vi "DAQ.vi"() -> (0 "Error Out":errorcluster)   [LabVIEW 2017]
uses:
  <vilib>/dex/Flush And Wait Empty Condition.ctl
  <vilib>/Platform/TimedLoop/XDataNode/timing_clust.ctl
  <vilib>/Platform/TimedLoop/XDataNode/nitl_modes.ctl
  <vilib>/Platform/TimedLoop/XDataNode/wakeup.ctl
  <vilib>/DAQmx/read.llb/DAQmx Read (Analog 1D DBL NChan 1Samp).vi
  <vilib>/DAQmx/miscellaneous.llb/DAQmx Fill In Error Info.vi
  <vilib>/Platform/TimedLoop/XDataNode/XDataNode.xnode
  <vilib>/Platform/TimedLoop/XDataNode/XDNodeRunTimeDep.lvlib
  <resource>/objmgr/ni.dex.rc
panel:
  out "Producer Loop Time":i64
  out "Consumer Loop Time":u32
  in  "Error In":errorcluster
  out "Time":dbl
  out "Available Elements for Writing":i32
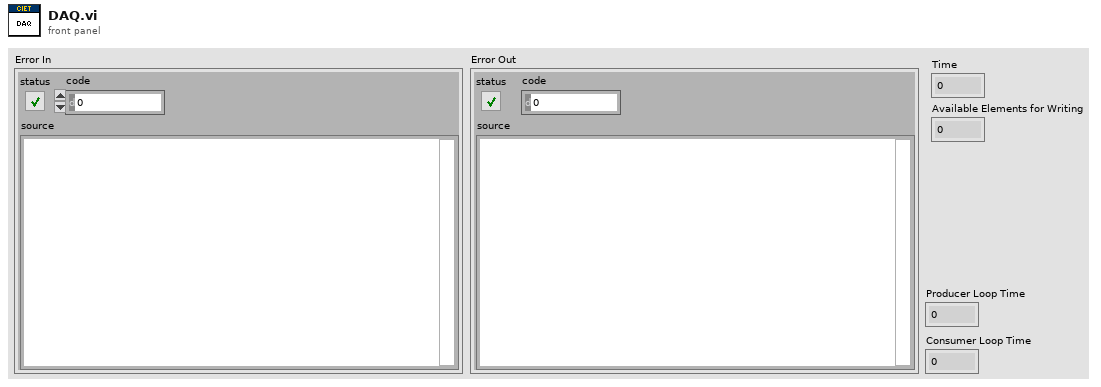
[diagram p1: front panel]
types:
  T1 = typedef "Flush And Wait Empty Condition.ctl" = u8
  T2 = typedef "XDNodeRunTimeDep.lvlib/timing_clust.ctl" = cluster{"Expected End [f-1]":u64, "Actual End [f-1]":u64, "Finished Late? [f-1]":bool, "Expected End [i-1]":u64, "Actual End [i-1]":u64, "Finished Late? [i-1]":bool, "Expected Start [i]":u64, "Actual Start [i]":u64, "Expected Start [f]":u64, "Actual Start [f]":u64, "Source Name":string, "Structure Name":string, "Period":i64, "Deadline":i64, "Offset":i64, "Start":i64, "Priority":i32, "Timeout":i32, "Mode":T3, "Wakeup Reason":T4, "Error":errorcluster, "Source Type":string, "Secondary Source Type":string, "Global End Time":u64, "Global Start Time":u64, "Frame Duration":u64, "Iteration Duration":u64, "Assigned CPU":i32, "I/O Scan Engine Mode":u32}
  T3 = typedef "XDNodeRunTimeDep.lvlib/nitl_modes.ctl" = enum32{"No Change", "Process missed periods, maintain original phase", "Discard missed periods, maintain original phase", "Process missed periods, ignore original phase", "Discard missed periods, ignore original phase"}
  T4 = typedef "XDNodeRunTimeDep.lvlib/wakeup.ctl" = enum32{"Normal", "Aborted", "Asynchronous wakeup", "Timing source error", "Timed loop error", "Timeout"}
  T5 = cluster{"[0]":sgl, "[1]":sgl, "[2]":sgl, "[3]":sgl, "[4]":sgl, "[5]":sgl, "[6]":sgl, "[7]":sgl, "[8]":sgl, "[9]":sgl, "[10]":sgl, "[11]":sgl, "[12]":sgl, "[13]":sgl, "[14]":sgl, "[15]":sgl, "[16]":sgl, "[17]":sgl, "[18]":sgl, "[19]":sgl, "[20]":sgl, "[21]":sgl, "[22]":sgl, "[23]":sgl, "[24]":sgl, "[25]":sgl, "[26]":sgl, "[27]":sgl, "[28]":sgl, "[29]":sgl, "[30]":sgl, "[31]":sgl, "[32]":sgl, "[33]":sgl, "[34]":sgl, "[35]":sgl, "[36]":sgl, "[37]":sgl, "[38]":sgl, "[39]":sgl, "[40]":sgl, "[41]":sgl, "[42]":sgl, "[43]":sgl, "[44]":sgl, "[45]":sgl, "[46]":sgl, "[47]":sgl, "[48]":sgl, "[49]":sgl, "[50]":sgl, "[51]":sgl, "[52]":sgl, "[53]":sgl, "[54]":sgl, "[55]":sgl, "[56]":sgl}
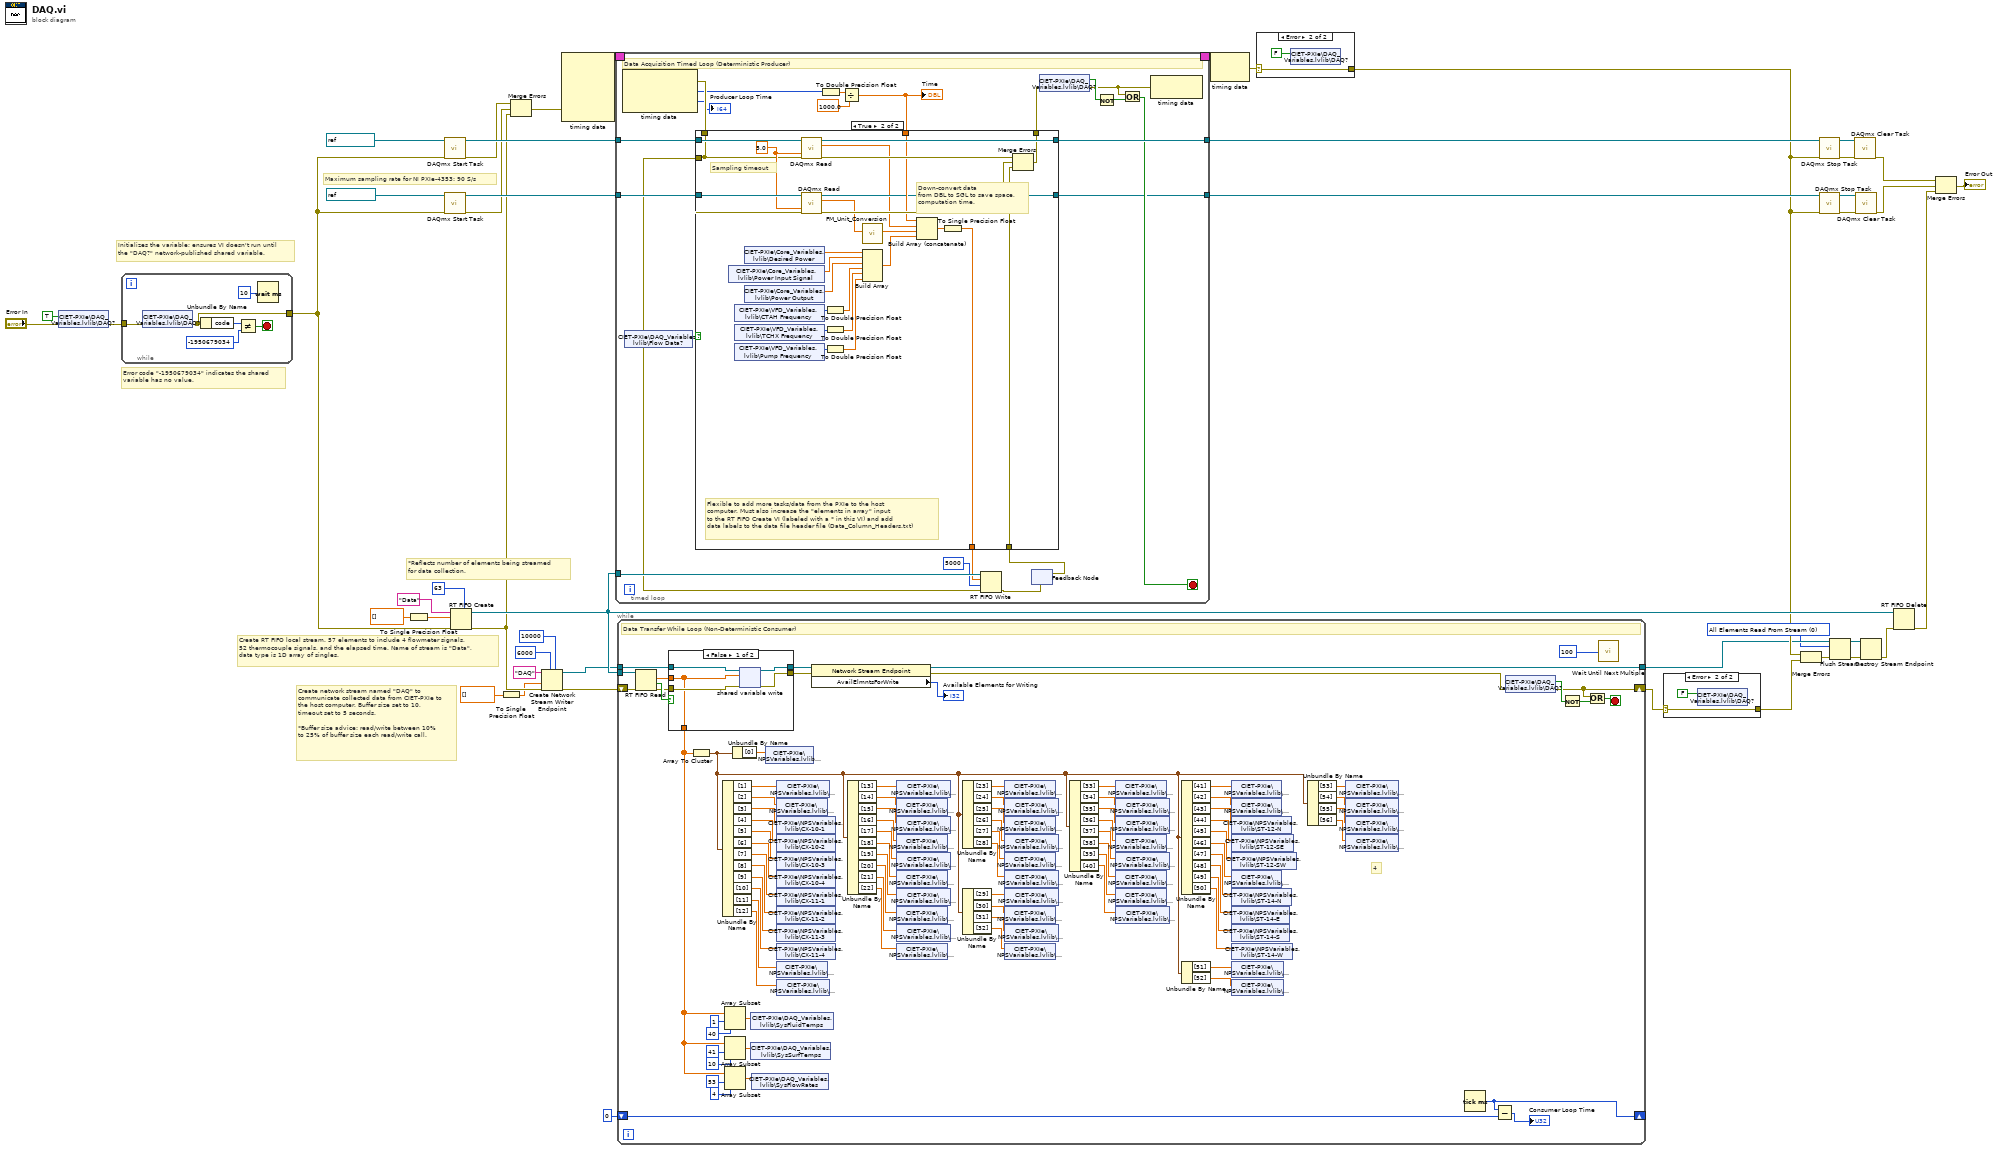
[diagram p0: block diagram]
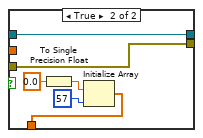
[diagram p4: hidden frame]
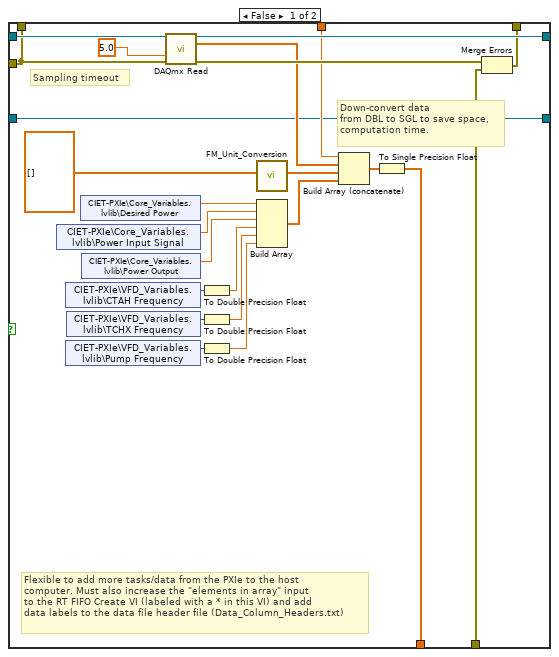
[diagram p5: hidden frame]
diagram:
  w3 = T1 0 items=["All Elements Read From Stream", "All Elements Available for Reading"] ("wait condition")
  # "*Reflects number of elements being streamed\nfor data collection."
  # "Create RT FIFO local stream. 57 elements to include 4 flowmeter signals,\n52 thermocouple signals, and the elapsed time. Name of stream is \"Data\",\ndata type is 1D array of singles."
  # "Create network stream named \"DAQ\" to communicate collected data from CIET-PXIe to the host computer. Buffer size set to 10, timeout set to 5 seconds. \n\n*Buffer size advice: read/write between 10%\nto 25% of buffer size each read/write call."
  # "Maximum sampling rate for NI PXIe-4353: 90 S/s"
  # "Initializes the variable; ensures VI doesn't run until\nthe \"DAQ?\" network-published shared variable."
  # "Error code \"-1950679034\" indicates the shared\nvariable has no value."
  n1 = shared-variable "CIET-PXIe\\DAQ_Variables.lvlib\\DAQ?"(TRUE ("Active?"), error in="Error In") -> (error out=w23:errorcluster)
  n2 = while {
    tunnel: w23 -> [w52]
    tunnel: [w51] -> w22
    stop <- w48 stop-if-true
    n3 = shared-variable "CIET-PXIe\\DAQ_Variables.lvlib\\DAQ?"(error in=w52) -> (error out=w51:errorcluster)  [unwired: 1 out]
    n4 = Unbundle By Name(w51) -> ("code"=w50:i32)
    n5 = Not Equal?(x=w50, y=-1950679034) -> (x != y?=w48:bool)
    n6 = Wait (ms)(milliseconds to wait=u32 10) -> ()  [unwired: 1 out]
  }
  n7 = To Single Precision Float(number=dbl[] []) -> (single precision float=w33:sgl[])
  n8 = call <vilib>:"DAQmx Start Task.vi"("task/channels in"=refnum<k21> "CIET-TC", "error in"=w22) -> ("task out"=w43:refnum<k21>, "error out"=w27:errorcluster)  [unwired: 12 in]
  n9 = call <vilib>:"DAQmx Start Task.vi"("task/channels in"=refnum<k21> "CIET-FM", "error in"=w22) -> ("task out"=w42:refnum<k21>, "error out"=w28:errorcluster)  [unwired: 12 in]
  n10 = RT FIFO Create(0:"Data" ("name (unnamed)"), 1:w33, 3:w22, 6:u32 63 ("elements in array (1)")) -> (8:w26:refnum<k33>, 11:w18:errorcluster)  [unwired: 4 in, 1 out]
  n11 = To Single Precision Float(number=dbl[] []) -> (single precision float=w8:sgl[])
  n12 = Merge Errors(w27, w28, w18) -> (w29:errorcluster)
  n13 = Create Network Stream Writer Endpoint(5:10000 ("timeout in ms (-1)"), 7:6000 ("writer buffer size"), 8:w18, 9:w8, 11:"DAQ" ("writer name")) -> (0:w19:errorcluster, 3:w17:refnum<k21>)  [unwired: 2 in]
  n14 = node-c288(w29) -> (w47:T2)  [unwired: 4 in]
  n15 = timed-loop {
    timing: w47 -> [_]
    timing-out: [_] -> w46
    tunnel: w26 -> [w72]
    tunnel: w43 -> [w75]
    tunnel: [w73] -> w37
    tunnel: w42 -> [w74]
    tunnel: [w60] -> w36
    stop <- w67 stop-if-true
    # "Data Acquisition Timed Loop (Deterministic Producer)"
    n16 = node-c288() -> (w70:errorcluster, w61:i64, →"Producer Loop Time":i64)  [unwired: 1 in]
    n17 = shared-variable "CIET-PXIe\\DAQ_Variables.lvlib\\Flow Data?"() -> (w55:bool)  [unwired: 1 in, 1 out]
    n18 = To Double Precision Float(number=w61) -> (double precision float=w64:dbl)
    n19 = Divide(x=w64, y=1000.0) -> (x/y=w63:dbl)
    "Time" <- w63
    n20 = feedback #1() -> (w56:errorcluster)  [unwired: 1 in]
    n21 = case shown="True" w55 {
      tunnel: w75 -> [w99 w125]
      tunnel: w74 -> [w79 w124]
      tunnel: [w97 w122] -> w73
      tunnel: [w95 w120] -> w58
      tunnel: w70 -> [w76 w100]
      tunnel: w56 -> [w77 w117]
      tunnel: [w93 w116] -> w66
      tunnel: w63 -> [w92 w115]
      tunnel: [w79 w114] -> w60
      tunnel: [w76 w100] -> w54
      frame False {
        # "Flexible to add more tasks/data from the PXIe to the host \ncomputer. Must also increase the \"elements in array\" input \nto the RT FIFO Create VI (labeled with a * in this VI) and add\ndata labels to the data file header file (Data_Column_Headers.txt)"
        # "Down-convert data\nfrom DBL to SGL to save space,\ncomputation time."
        # "Sampling timeout"
        n22 = shared-variable "CIET-PXIe\\Core_Variables.lvlib\\Power Input Signal"() -> (w82:dbl)  [unwired: 1 in, 1 out]
        n23 = shared-variable "CIET-PXIe\\VFD_Variables.lvlib\\CTAH Frequency"() -> (w84:u16)  [unwired: 1 in, 1 out]
        n24 = shared-variable "CIET-PXIe\\VFD_Variables.lvlib\\Pump Frequency"() -> (w86:u16)  [unwired: 1 in, 1 out]
        n25 = shared-variable "CIET-PXIe\\VFD_Variables.lvlib\\TCHX Frequency"() -> (w85:u16)  [unwired: 1 in, 1 out]
        n26 = shared-variable "CIET-PXIe\\Core_Variables.lvlib\\Desired Power"() -> (w81:dbl)  [unwired: 1 in, 1 out]
        n27 = shared-variable "CIET-PXIe\\Core_Variables.lvlib\\Power Output"() -> (w83:dbl)  [unwired: 1 in, 1 out]
        n28 = call-poly <vilib>:"DAQmx Read.vi"("task/channels in"=w99, "timeout"=5.0, "error in"=w76) -> ("task out"=w97:refnum<k21>, "data"=w91:dbl[], "error out"=w94:errorcluster)  [unwired: 10 in]
        n29 = To Double Precision Float(number=w84) -> (double precision float=w87:dbl)
        n30 = To Double Precision Float(number=w85) -> (double precision float=w88:dbl)
        n31 = To Double Precision Float(number=w86) -> (double precision float=w89:dbl)
        n32 = call "FM_Unit_Conversion.vi"("Input Array [A]"=dbl[] []) -> ("Output Array [kg/h]"=w90:dbl[])  [unwired: 10 in]
        n33 = Build Array(w81, w82, w83, w87, w88, w89) -> (w80:dbl[])
        n34 = Build Array (concatenate)(w92, w91, w90, w80) -> (w96:dbl[])
        n35 = To Single Precision Float(number=w96) -> (single precision float=w95:sgl[])
        n36 = Merge Errors(w94, w77) -> (w93:errorcluster)
      }
      frame True {
        w123 = 5.0 ("timeout")
        # "Flexible to add more tasks/data from the PXIe to the host \ncomputer. Must also increase the \"elements in array\" input \nto the RT FIFO Create VI (labeled with a * in this VI) and add\ndata labels to the data file header file (Data_Column_Headers.txt)"
        # "Down-convert data\nfrom DBL to SGL to save space,\ncomputation time."
        # "Sampling timeout"
        n37 = shared-variable "CIET-PXIe\\Core_Variables.lvlib\\Power Input Signal"() -> (w103:dbl)  [unwired: 1 in, 1 out]
        n38 = shared-variable "CIET-PXIe\\VFD_Variables.lvlib\\CTAH Frequency"() -> (w105:u16)  [unwired: 1 in, 1 out]
        n39 = shared-variable "CIET-PXIe\\VFD_Variables.lvlib\\Pump Frequency"() -> (w107:u16)  [unwired: 1 in, 1 out]
        n40 = shared-variable "CIET-PXIe\\VFD_Variables.lvlib\\TCHX Frequency"() -> (w106:u16)  [unwired: 1 in, 1 out]
        n41 = shared-variable "CIET-PXIe\\Core_Variables.lvlib\\Desired Power"() -> (w102:dbl)  [unwired: 1 in, 1 out]
        n42 = shared-variable "CIET-PXIe\\Core_Variables.lvlib\\Power Output"() -> (w104:dbl)  [unwired: 1 in, 1 out]
        n43 = call-poly <vilib>:"DAQmx Read.vi"("task/channels in"=w125, "timeout"=w123, "error in"=w100) -> ("task out"=w122:refnum<k21>, "data"=w113:dbl[], "error out"=w118:errorcluster)  [unwired: 10 in]
        n44 = call-poly <vilib>:"DAQmx Read.vi"("task/channels in"=w124, "timeout"=w123, "error in"=w100) -> ("task out"=w114:refnum<k21>, "data"=w111:dbl[], "error out"=w119:errorcluster)  [unwired: 10 in]
        n45 = To Double Precision Float(number=w105) -> (double precision float=w108:dbl)
        n46 = To Double Precision Float(number=w106) -> (double precision float=w109:dbl)
        n47 = To Double Precision Float(number=w107) -> (double precision float=w110:dbl)
        n48 = call "FM_Unit_Conversion.vi"("Input Array [A]"=w111) -> ("Output Array [kg/h]"=w112:dbl[])  [unwired: 10 in]
        n49 = Build Array(w102, w103, w104, w108, w109, w110) -> (w101:dbl[])
        n50 = Build Array (concatenate)(w115, w113, w112, w101) -> (w121:dbl[])
        n51 = To Single Precision Float(number=w121) -> (single precision float=w120:sgl[])
        n52 = Merge Errors(w118, w119, w117) -> (w116:errorcluster)
      }
    }
    n53 = RT FIFO Write(0:w72, 1:w58, 2:5000 ("timeout in ms (0)"), 3:w54) -> (11:w57:errorcluster)  [unwired: 1 in, 3 out]
    n54 = feedback-in #1(w57) -> ()
    n55 = shared-variable "CIET-PXIe\\DAQ_Variables.lvlib\\DAQ?"(error in=w66) -> (w69:bool, error out=w65:errorcluster)
    n56 = Not(x=w69) -> (.not. x?=w68:bool)
    n57 = Or(x=w65, y=w68) -> (x .or. y?=w67:bool)
    n58 = node-c288(w65) -> ()  [unwired: 1 out]
  }
  n59 = while {
    tunnel: w26 -> [w219]
    shift-right: [w208] -> w20
    shift-left: w19 -> [w218]
    tunnel: w17 -> [w210]
    tunnel: [w205] -> w10
    shift-right: [w145] -> _
    shift-left: u32 0 ("millisecond timer value") -> [w144]
    stop <- w211 stop-if-true
    # "4"
    # "Data Transfer While Loop (Non-Deterministic Consumer)"
    n60 = RT FIFO Read(0:w219, 3:w218) -> (9:w215:sgl[], 10:w216:bool, 11:w214:errorcluster)  [unwired: 2 in, 2 out]
    n61 = case shown="False" w216 {
      tunnel: w215 -> [w220 _]
      tunnel: w214 -> [w224 w230]
      tunnel: [w223 w230] -> w207
      tunnel: w210 -> [w222 w229]
      tunnel: [w221 w229] -> w206
      tunnel: [w220 w225] -> w136
      frame False {
        n62 = shared-variable-write(w222, w224, w220) -> (w221:refnum<k21>, w223:errorcluster)  [unwired: 1 in, 1 out]
      }
      frame True {
        n63 = To Single Precision Float(number=sgl 0.0) -> (single precision float=w228:sgl)
        n64 = Initialize Array(w228, 57 ("dimension size")) -> (w225:sgl[])
      }
    }
    n65 = Array To Cluster(array=w136) -> (cluster=w146:T5)
    n66 = Unbundle By Name(w146) -> ("[1]"=w202:sgl, "[2]"=w201:sgl, "[3]"=w200:sgl, "[4]"=w199:sgl, "[5]"=w198:sgl, "[6]"=w197:sgl, "[7]"=w196:sgl, "[8]"=w195:sgl, "[9]"=w194:sgl, "[10]"=w193:sgl, "[11]"=w192:sgl, "[12]"=w191:sgl)
    n67 = Array Subset(array=w136, index=1, length=40) -> (w140:sgl[])
    n68 = Array Subset(array=w136, index=41, length=10) -> (w138:sgl[])
    n69 = Array Subset(array=w136, index=53, length=4) -> (w133:sgl[])
    n70 = Unbundle By Name(w146) -> ("[0]"=w203:sgl)
    n71 = shared-variable "CIET-PXIe\\DAQ_Variables.lvlib\\SysFluidTemps"(w140) -> ()  [unwired: 1 in, 1 out]
    n72 = shared-variable "CIET-PXIe\\DAQ_Variables.lvlib\\SysSurfTemps"(w138) -> ()  [unwired: 1 in, 1 out]
    n73 = shared-variable "CIET-PXIe\\DAQ_Variables.lvlib\\SysFlowRates"(w133) -> ()  [unwired: 1 in, 1 out]
    n74 = shared-variable "CIET-PXIe\\NPSVariables.lvlib\\Time"(w203) -> ()  [unwired: 1 in, 1 out]
    n75 = shared-variable "CIET-PXIe\\NPSVariables.lvlib\\WT-10"(w202) -> ()  [unwired: 1 in, 1 out]
    n76 = shared-variable "CIET-PXIe\\NPSVariables.lvlib\\BT-11"(w201) -> ()  [unwired: 1 in, 1 out]
    n77 = shared-variable "CIET-PXIe\\NPSVariables.lvlib\\CX-10-1"(w200) -> ()  [unwired: 1 in, 1 out]
    n78 = shared-variable "CIET-PXIe\\NPSVariables.lvlib\\CX-10-2"(w199) -> ()  [unwired: 1 in, 1 out]
    n79 = shared-variable "CIET-PXIe\\NPSVariables.lvlib\\CX-10-3"(w198) -> ()  [unwired: 1 in, 1 out]
    n80 = shared-variable "CIET-PXIe\\NPSVariables.lvlib\\CX-10-4"(w197) -> ()  [unwired: 1 in, 1 out]
    n81 = shared-variable "CIET-PXIe\\NPSVariables.lvlib\\CX-11-1"(w196) -> ()  [unwired: 1 in, 1 out]
    n82 = shared-variable "CIET-PXIe\\NPSVariables.lvlib\\CX-11-2"(w195) -> ()  [unwired: 1 in, 1 out]
    n83 = shared-variable "CIET-PXIe\\NPSVariables.lvlib\\CX-11-3"(w194) -> ()  [unwired: 1 in, 1 out]
    n84 = shared-variable "CIET-PXIe\\NPSVariables.lvlib\\CX-11-4"(w193) -> ()  [unwired: 1 in, 1 out]
    n85 = shared-variable "CIET-PXIe\\NPSVariables.lvlib\\BT-12"(w192) -> ()  [unwired: 1 in, 1 out]
    n86 = shared-variable "CIET-PXIe\\NPSVariables.lvlib\\WT-13"(w191) -> ()  [unwired: 1 in, 1 out]
    n87 = property class="Network Stream Endpoint"(reference=w206, error in=w207) -> (reference out=w205:refnum<k21>, error out=w204:errorcluster, "AvailElmntsForWrite"=→"Available Elements for Writing":i32)
    n88 = Unbundle By Name(w146) -> ("[13]"=w190:sgl, "[14]"=w189:sgl, "[15]"=w188:sgl, "[16]"=w187:sgl, "[17]"=w186:sgl, "[18]"=w185:sgl, "[19]"=w184:sgl, "[20]"=w183:sgl, "[21]"=w182:sgl, "[22]"=w181:sgl)
    n89 = shared-variable "CIET-PXIe\\NPSVariables.lvlib\\WT-20"(w190) -> ()  [unwired: 1 in, 1 out]
    n90 = shared-variable "CIET-PXIe\\NPSVariables.lvlib\\BT-21"(w189) -> ()  [unwired: 1 in, 1 out]
    n91 = shared-variable "CIET-PXIe\\NPSVariables.lvlib\\WT-22"(w188) -> ()  [unwired: 1 in, 1 out]
    n92 = shared-variable "CIET-PXIe\\NPSVariables.lvlib\\BT-23"(w187) -> ()  [unwired: 1 in, 1 out]
    n93 = shared-variable "CIET-PXIe\\NPSVariables.lvlib\\WT-24"(w186) -> ()  [unwired: 1 in, 1 out]
    n94 = shared-variable "CIET-PXIe\\NPSVariables.lvlib\\BT-25"(w185) -> ()  [unwired: 1 in, 1 out]
    n95 = shared-variable "CIET-PXIe\\NPSVariables.lvlib\\WT-26"(w184) -> ()  [unwired: 1 in, 1 out]
    n96 = shared-variable "CIET-PXIe\\NPSVariables.lvlib\\BT-27"(w183) -> ()  [unwired: 1 in, 1 out]
    n97 = shared-variable "CIET-PXIe\\NPSVariables.lvlib\\WT-28"(w182) -> ()  [unwired: 1 in, 1 out]
    n98 = shared-variable "CIET-PXIe\\NPSVariables.lvlib\\BT-29"(w181) -> ()  [unwired: 1 in, 1 out]
    n99 = Unbundle By Name(w146) -> ("[23]"=w180:sgl, "[24]"=w179:sgl, "[25]"=w178:sgl, "[26]"=w177:sgl, "[27]"=w176:sgl, "[28]"=w175:sgl)
    n100 = Unbundle By Name(w146) -> ("[29]"=w174:sgl, "[30]"=w173:sgl, "[31]"=w172:sgl, "[32]"=w171:sgl)
    n101 = shared-variable "CIET-PXIe\\NPSVariables.lvlib\\BT-30"(w180) -> ()  [unwired: 1 in, 1 out]
    n102 = shared-variable "CIET-PXIe\\NPSVariables.lvlib\\WT-31"(w179) -> ()  [unwired: 1 in, 1 out]
    n103 = shared-variable "CIET-PXIe\\NPSVariables.lvlib\\BT-32"(w178) -> ()  [unwired: 1 in, 1 out]
    n104 = shared-variable "CIET-PXIe\\NPSVariables.lvlib\\WT-33"(w177) -> ()  [unwired: 1 in, 1 out]
    n105 = shared-variable "CIET-PXIe\\NPSVariables.lvlib\\BT-34"(w176) -> ()  [unwired: 1 in, 1 out]
    n106 = shared-variable "CIET-PXIe\\NPSVariables.lvlib\\WT-35"(w175) -> ()  [unwired: 1 in, 1 out]
    n107 = shared-variable "CIET-PXIe\\NPSVariables.lvlib\\WT-40"(w174) -> ()  [unwired: 1 in, 1 out]
    n108 = shared-variable "CIET-PXIe\\NPSVariables.lvlib\\BT-41"(w173) -> ()  [unwired: 1 in, 1 out]
    n109 = shared-variable "CIET-PXIe\\NPSVariables.lvlib\\WT-42"(w172) -> ()  [unwired: 1 in, 1 out]
    n110 = shared-variable "CIET-PXIe\\NPSVariables.lvlib\\BT-43"(w171) -> ()  [unwired: 1 in, 1 out]
    n111 = Unbundle By Name(w146) -> ("[33]"=w170:sgl, "[34]"=w169:sgl, "[35]"=w168:sgl, "[36]"=w167:sgl, "[37]"=w166:sgl, "[38]"=w165:sgl, "[39]"=w164:sgl, "[40]"=w163:sgl)
    n112 = shared-variable "CIET-PXIe\\NPSVariables.lvlib\\BT-60"(w170) -> ()  [unwired: 1 in, 1 out]
    n113 = shared-variable "CIET-PXIe\\NPSVariables.lvlib\\WT-61"(w169) -> ()  [unwired: 1 in, 1 out]
    n114 = shared-variable "CIET-PXIe\\NPSVariables.lvlib\\WT-62"(w168) -> ()  [unwired: 1 in, 1 out]
    n115 = shared-variable "CIET-PXIe\\NPSVariables.lvlib\\BT-63"(w167) -> ()  [unwired: 1 in, 1 out]
    n116 = shared-variable "CIET-PXIe\\NPSVariables.lvlib\\WT-64"(w166) -> ()  [unwired: 1 in, 1 out]
    n117 = shared-variable "CIET-PXIe\\NPSVariables.lvlib\\BT-65"(w165) -> ()  [unwired: 1 in, 1 out]
    n118 = shared-variable "CIET-PXIe\\NPSVariables.lvlib\\BT-66"(w164) -> ()  [unwired: 1 in, 1 out]
    n119 = shared-variable "CIET-PXIe\\NPSVariables.lvlib\\WT-67"(w163) -> ()  [unwired: 1 in, 1 out]
    n120 = Unbundle By Name(w146) -> ("[41]"=w162:sgl, "[42]"=w161:sgl, "[43]"=w160:sgl, "[44]"=w159:sgl, "[45]"=w158:sgl, "[46]"=w157:sgl, "[47]"=w156:sgl, "[48]"=w155:sgl, "[49]"=w154:sgl, "[50]"=w153:sgl)
    n121 = Unbundle By Name(w146) -> ("[51]"=w152:sgl, "[52]"=w151:sgl)
    n122 = shared-variable "CIET-PXIe\\NPSVariables.lvlib\\ST-10"(w162) -> ()  [unwired: 1 in, 1 out]
    n123 = shared-variable "CIET-PXIe\\NPSVariables.lvlib\\ST-11"(w161) -> ()  [unwired: 1 in, 1 out]
    n124 = shared-variable "CIET-PXIe\\NPSVariables.lvlib\\ST-12-N"(w160) -> ()  [unwired: 1 in, 1 out]
    n125 = shared-variable "CIET-PXIe\\NPSVariables.lvlib\\ST-12-SE"(w159) -> ()  [unwired: 1 in, 1 out]
    n126 = shared-variable "CIET-PXIe\\NPSVariables.lvlib\\ST-12-SW"(w158) -> ()  [unwired: 1 in, 1 out]
    n127 = shared-variable "CIET-PXIe\\NPSVariables.lvlib\\ST-13"(w157) -> ()  [unwired: 1 in, 1 out]
    n128 = shared-variable "CIET-PXIe\\NPSVariables.lvlib\\ST-14-N"(w156) -> ()  [unwired: 1 in, 1 out]
    n129 = shared-variable "CIET-PXIe\\NPSVariables.lvlib\\ST-14-E"(w155) -> ()  [unwired: 1 in, 1 out]
    n130 = shared-variable "CIET-PXIe\\NPSVariables.lvlib\\ST-14-S"(w154) -> ()  [unwired: 1 in, 1 out]
    n131 = shared-variable "CIET-PXIe\\NPSVariables.lvlib\\ST-14-W"(w153) -> ()  [unwired: 1 in, 1 out]
    n132 = shared-variable "CIET-PXIe\\NPSVariables.lvlib\\AT-01"(w152) -> ()  [unwired: 1 in, 1 out]
    n133 = shared-variable "CIET-PXIe\\NPSVariables.lvlib\\AT-02"(w151) -> ()  [unwired: 1 in, 1 out]
    n134 = Unbundle By Name(w146) -> ("[53]"=w150:sgl, "[54]"=w149:sgl, "[55]"=w148:sgl, "[56]"=w147:sgl)
    n135 = shared-variable "CIET-PXIe\\NPSVariables.lvlib\\FM-20"(w150) -> ()  [unwired: 1 in, 1 out]
    n136 = shared-variable "CIET-PXIe\\NPSVariables.lvlib\\FM-30"(w149) -> ()  [unwired: 1 in, 1 out]
    n137 = shared-variable "CIET-PXIe\\NPSVariables.lvlib\\FM-40"(w148) -> ()  [unwired: 1 in, 1 out]
    n138 = shared-variable "CIET-PXIe\\NPSVariables.lvlib\\FM-60"(w147) -> ()  [unwired: 1 in, 1 out]
    n139 = Tick Count (ms)() -> (millisecond timer value=w145:u32)
    n140 = Subtract(x=w145, y=w144) -> (x-y=→"Consumer Loop Time":u32)
    n141 = shared-variable "CIET-PXIe\\DAQ_Variables.lvlib\\DAQ?"(error in=w204) -> (w213:bool, error out=w208:errorcluster)
    n142 = Not(x=w213) -> (.not. x?=w212:bool)
    n143 = Or(x=w208, y=w212) -> (x .or. y?=w211:bool)
    n144 = call "Wait Until Next Multiple"("Count(mSec)"=u32 100) -> ()  [unwired: 1 out]
  }
  n145 = node-c288(w46) -> (w21:errorcluster)
  n146 = case shown="Error" w21 {
    selector: w21 -> [w231 w232]
    tunnel: [w231 w232] -> w16
    frame No Error {
    }
    frame Error {
      n147 = shared-variable "CIET-PXIe\\DAQ_Variables.lvlib\\DAQ?"(FALSE ("DAQ?")) -> ()  [unwired: 1 in, 1 out]
    }
  }
  n148 = case shown="Error" w20 {
    selector: w20 -> [w234 w235]
    tunnel: [w234 w235] -> w15
    frame No Error {
    }
    frame Error {
      n149 = shared-variable "CIET-PXIe\\DAQ_Variables.lvlib\\DAQ?"(FALSE ("DAQ?")) -> ()  [unwired: 1 in, 1 out]
    }
  }
  n150 = Merge Errors(w16, w15) -> (w12:errorcluster)
  n151 = call <vilib>:"DAQmx Stop Task.vi"("task/channels in"=w37, "error in"=w16) -> ("task out"=w40:refnum<k21>, "error out"=w41:errorcluster)  [unwired: 12 in]
  n152 = call <vilib>:"DAQmx Stop Task.vi"("task/channels in"=w36, "error in"=w16) -> ("task out"=w38:refnum<k21>, "error out"=w39:errorcluster)  [unwired: 12 in]
  n153 = Flush Stream(8:w12, 10:w3, 11:w10) -> (0:w14:errorcluster, 3:w13:refnum<k21>)  [unwired: 1 in, 1 out]
  n154 = call <vilib>:"DAQmx Clear Task.vi"("task in"=w40, "error in"=w41) -> ("error out"=w35:errorcluster)  [unwired: 13 in]
  n155 = call <vilib>:"DAQmx Clear Task.vi"("task in"=w38, "error in"=w39) -> ("error out"=w34:errorcluster)  [unwired: 13 in]
  n156 = Destroy Stream Endpoint(8:w14, 11:w13) -> (0:w11:errorcluster)
  n157 = RT FIFO Delete(0:w26, 3:w11) -> (11:w5:errorcluster)  [unwired: 1 in]
  n158 = Merge Errors(w35, w34, w5) -> (→"Error Out":errorcluster)
